vi "Station.Home.Check.vi"(8 "error in (no error)":errorcluster) -> (0 "error out":errorcluster, 1 "Homed?":bool, 2 "Error?":bool, 3 "Statuses":T2[](array[typedef]), 5 "Station Home Status":T1)   [LabVIEW 2016]
uses:
  Station.Home.Status.ctl
  Station.Home.Status.Bits.ctl
  tools/Translator/Translator.Message.ctl
  Drivers/FestoCPX/FestoCPX.State.ctl
  Drivers/V7310/LowLevel/V7310.LaserStatus.ctl
  Drivers/V7310/V7310.Data.Status.State.ctl
  Drivers/Keyence/Keyence.Data.Status.State.ctl
  tools/Translator/Translator.FormatMessage.vi
  tools/Translator/Translator.Global.vi
  Global/ApplicationGlobal.vi
  Sequence/Sequence.Global.vi
  Drivers/FestoCPX/FestoCPX.Global.vi
  Drivers/V7310/LowLevel/V7310.Global.vi
  Drivers/Keyence/LowLevel/Keyence.Global.vi
  Station.Global.vi
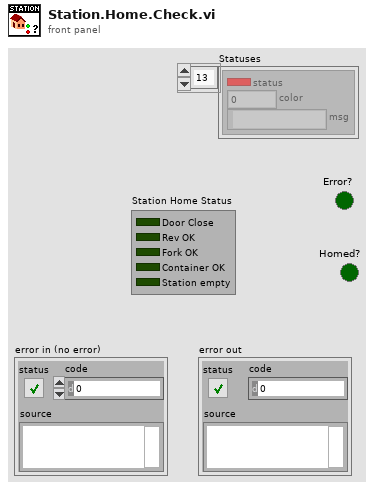
[diagram p1: front panel]
types:
  T1 = typedef "Station.Home.Status.Bits.ctl" = cluster{"Door Close":bool, "Rev OK":bool, "Fork OK":bool, "Container OK":bool, "Station empty":bool}
  T2 = typedef "Station.Home.Status.ctl" = cluster{"status":bool, "color":u32, "msg":string}
  T3 = typedef "Translator.Message.ctl" = enum16{"-", "Event confirmed", "Log out", "Log in", "Shutdown", "Cancel", "Start", "Begin time", "End time", "Duration", "Service Mode", "Ignore Results", "Serial Format", "On", "Off", "OK", "NOK", "NOK %s", "Home", "Work", "Close", "Open", "In progress...", "Missing", "Empty", "Hardware failure", "Initial", "Default", "Total", "Out of range", "Free disk space is below 1GB - contact technician", "Error %d >> %s", "Error %d >> %s >> %s", "Msg %d >> %s", "Laser msg %d %s", "Laser cmd error %s %d", "Laser cmd failed %s", "Laser cmd warning %s", "Laser disconnected", "Laser status %s", "Laser already started", "Laser job unkonwn %s", "Laser job missing %s", "Laser job select failure %s", "Unable to start laser printing (%s)", "Unable to stop laser printing (%s)", "Laser marking aborted", "Laser marking timeout", "Unable to reset Laser Interlock (%s)", "Unable to trigger Laser. Laser not ready (%s)", "Laser job '%s' coordinates not configured", "Starting %s", "Quitting %s", "Configured", "Initializing", "Quitting", "Loading", "Loaded %d results", "Loaded %d events", "Running", "Stopped", "Summary", "Laser", "Do you want to continue?", "Do you want to delete the configuration?", "The configuration is being used by an order. Unable to delete!", "Press confirm button", "Station is not based. Do you want to exit?", "Station requires changeover. Do you want to run the test?", "Test options are not set as default. Do you want to continue?", "Formatting of WabcoNo is disabled. Do you want to continue?", "Product not detected. Do you want to continue?", "Product scan failed. Do you want to continue?", "Calibration", "Log out?", "System", "All", "IDLE", "Translating...%s", "Not found", "Alarm %s", "Run", "Skip", "Abort", "Repeat", "Please wait...", "Database disconnected", "Database disconnected - changeover disabled!", "Login to database successful", "Login to database failed: %d; %s", "Unable to check the product status of reference %d - database disconnected", "Unable to set the product status of reference %d - database disconnected", "Variant file backup %s", "Read variant (%s)", "Result", "Station armed!", "Station requires changeover!", "Select reference number...", "EMERGENCY BUTTON - press Control button", "EMERGENCY DOOR - press Control button", "Resetting Emergency...", "Unable to reset safety circuit - Emergency Button pressed", "Unable to reset safety circuit - Emergency Side Door open", "Station not based", "Station based", "Station not empty", "Station basing...", "No order", "Press Start to begin new order", "Scanning new order", "Order NOK. Correct or scan again", "Order OK. Press Accept", "Order ready", "Revolver incorrect", "Fork incorrect", "Revolver missing", "Revolver empty", "Container missing", "Offline results", "Offline statistics", "Updating statistics %.1f %%", "DMC Configurator", "Door open", "Close the front door", "Press start button", "Done. Open the front door", "Running...", "Running...%.1f %%", "Pause %s", "Pause %s. NOK container missing", "Pause %s. OK container missing", "Pause %s. Revolver empty", "Pause %s. Revolver missing", "Pause %s. Revolver incorrect", "Pause %s. Fork missing", "Pause %s. Fork incorrect", "Pause %s. Too many failures", "Pause %s. Unloading failure", "Pause %s. One slot is not working", "Pause %s. Part order is done. Empty OK container", "Pause %s. Unable to move product to slot", "Pause %s. Unable to move back product pusher", "Pause %s. Unable to lift product", "Pause %s. Unable to move back product lifter", "Pause %s. Unable to move product arm to Work", "Pause %s. Unable to move product arm to NOK", "Pause %s. Unable to move product arm to OK", "Pause %s. Unable to unsuck the NOK product", "Pause %s. Unable to drop the NOK product", "Pause %s. Product OK missing", "Pause %s. Unable to unsuck the OK product", "Pause %s. Unable to drop the OK product", "Stopping...", "File '%s' is missing", "File '%s' is broken", "File '%s' is running", "Log file started (%s)", "Log file ended (%s)", "Log file stopped (%s)", "Log file ignored (%s)", "Log file exported (%s)", "Log file export failed (%s)", "Wrong serial number in log file", "Wrong reference number in log file", "Test steps are missing", "%s = %.3f", "Process param '%s' not found in DB", "Process param '%s' wrong order", "Process param '%s' value %.3f out of limits (%.3f; %.3f)", "Step%d param '%s' not found in DB", "Step%d param '%s' wrong order", "Step%d param '%s' value %.3f out of limits (%.3f; %.3f)", "Step%d EV '%s' not found in DB", "Step%d EV '%s' wrong order", "\"%s\" not found in DB", "\"%s\" wrong order", "\"%s\" value %.3f out of limits (%.3f; %.3f)", "\"%s\" not found in software", "Process init (%s)", "Process started", "Process restarted", "Process run", "Process done", "Process done - remove OK container", "Process aborted", "Process aborted at work", "Process aborted at home", "Process error", "Process error at home", "Process error at work", "Process close", "Process pause", "Process continue", "Process door open", "Process door close", "Process pause at slot %s due to %s", "Select plate from the order to process", "Do you want to start the process?", "Do you want to continue the process?", "There is unfinished order. Do you want to put the new order?", "Product %s %d OK", "Product %s %d NOK", "Unable to unload the slot %s. Product missing in the slot", "Unable to unload the slot %s. Product already in the arm", "Unable to accept the product as OK. Product missing in slot %s", "Unable to accept the product as OK. Product could not drop into the container at slot %s", "Unable to accept the product as NOK. Product could not drop into the container at slot %s", "Scan failed. Error %s", "Scan failed. Scanner disconnected", "Scan failed. Wrong Wabco number %d, limit (%d,%d)", "Scan failed. Wrong serial number %d, limit (%d,%d)", "Scan failed. Wrong date %d, limit (%d,%d)", "Scan failed. Wrong product wabco number %d (expected %d)", "Scan failed. Wrong product serial number %d (expected > 0)", "Scan OK %s", "Scan failed. Unable to determine table position (%s)", "Scan failed. Timeout", "Tune failed. Scanner disconnected", "Tune failed. Timeout", "%s = %d", "%s = %d->%d", "Unable to set %s = %.2f - Air Pressure Inside off", "Unable to set digital output '%s' = %d", "Unable to activate air pressure inside - timeout", "Unable to activate air pressure inside - aborted", "Unable to switch on Air Main Valve - Air Pressure Inlet off", "Unable to switch on Air Main Valve - Door open", "Unable to switch off Air Main Valve - timeout", "Unable to switch off Air Main Valve - aborted", "Unable to rotate Table - timeout", "Unable to rotate Table - aborted", "Unable to rotate Table - Product Move not in Home position", "Unable to rotate Table - Air Pressure Inside off", "Unable to rotate Table - Product Lift A not in Home position", "Unable to rotate Table - Product Lift B not in Home position", "Unable to rotate Table - unlock before movement timeout", "Unable to rotate Table - lock after movement timeout", "Unable to move Table Lock to %s position - timeout", "Unable to move Table Lock to %s position - aborted", "Unable to move Table Lock to %s position - Air Pressure Inside off", "Unable to move Table Lock to %s position - Table not in position", "Unable to move Product Lift A to %s position - timeout", "Unable to move Product Lift B to %s position - timeout", "Unable to move Product Lift A to %s position - aborted", "Unable to move Product Lift B to %s position - aborted", "Unable to move Product Lift A to %s position - Air Pressure Inside off", "Unable to move Product Lift B to %s position - Air Pressure Inside off", "Unable to move Product Lift A to %s position - Table not locked", "Unable to move Product Lift B to %s position - Table not locked", "Unable to move Product Lift A to %s position - Product Arm not in Work position", "Unable to move Product Lift B to %s position - Product Arm not in Work position", "Unable to set Product Suction Gripper %s to %s - timeout", "Unable to set Product Suction Gripper %s to %s - aborted", "Unable to set Product Suction Gripper %s to %s - Air Pressure Inside off", "Unable to set Product Suction Gripper %s to %s - Table slot unkown", "Unable to move Product Arm to %s position - timeout", "Unable to move Product Arm to %s position - aborted", "Unable to move Product Arm to %s position - Air Pressure Inside off", "Unable to move Product Arm to %s position - Product Lift A not in Home position", "Unable to move Product Arm to %s position - Product Lift B not in Home position", "Unable to move Product to %s position - timeout", "Unable to move Product to %s position - aborted", "Unable to move Product to %s position - Air Pressure Inside off", "Unable to move Product to %s position - Table not in position"}
  T4 = typedef "Sequence.Data.ctl" = cluster{"BeginTS":timestamp, "EndTS":timestamp, "State":T5, "Status.Work":T6, "Status.Process":T6, "Status.Home":T6, "Status.Wabco":T6, "Status.Client":T6, "BreakReason":T7, "BreakSource":T8, "DoorLock":bool, "Status.Prod":T9[], "UserAction":T13, "UserData":T14, "Error":errorcluster, "Code":T17, "Rotations":i32, "ProdIdx":i32, "ProdDone":T9[], "PrintedSerials-Wabco":i32[], "PrintedSerials-Client":i32[], "Counters-Wabco":T24, "Counters-Client":T24}
  T5 = typedef "Sequence.State.ctl" = enum16{"Init", "Idle", "Home", "Work", "Run", "Pause"}
  T6 = typedef "Sequence.Step.Status.ctl" = enum16{"-", "Pending", "Running", "Skipped", "Passed", "Failed", "Done", "Error", "Aborted", "Stopped"}
  T7 = typedef "Sequence.Test.BreakReason.ctl" = enum16{"-", "NOK container", "OK container", "Rev empty", "Rev missing", "Rev wrong", "Fork missing", "Fork wrong", "NOK limit", "Unload failure", "Single slot", "Part done", "Err: Prod move work", "Err: Prod move home", "Err: Prod lift work", "Err: Prod lift home", "Err: Prod Arm Work", "Err: Prod Arm NOK", "Err: Prod Arm OK", "Err: Prod NOK suck", "Err: Prod NOK drop", "Err: Prod OK missing", "Err: Prod OK suck", "Err: Prod OK drop"}
  T8 = typedef "Sequence.Test.BreakSource.ctl" = enum16{"-", "A", "B", "A/B"}
  T9 = typedef "Sequence.Test.Status.ctl" = cluster{"Slot":T10, "A":T12, "B":T12}
  T10 = typedef "Sequence.Slot.StatusData.ctl" = cluster{"ID":i32, "Unload":T11, "TS":timestamp, "duration":u32}
  T11 = typedef "Sequence.Test.Unload.Status.ctl" = enum16{"init", "check NOK", "check OK", "wait on NOK", "wait on OK", "wait on Unload", "done"}
  T12 = typedef "Sequence.Prod.StatusData.ctl" = cluster{"status":T6, "pause":T7, "present":bool, "printed":bool, "scanned":bool, "tuned":bool, "removed":bool, "LaserVariables":string[], "ScanerReadOut":string, "path":path, "corners":cluster{"X":i32, "Y":i32}[], "verification":u8}
  T13 = typedef "Sequence.UserActions.ctl" = cluster{"Stop":bool, "Pause":bool, "Next":bool}
  T14 = typedef "Sequence.UserData.ctl" = cluster{"GuiMode":T15, "Test":T16, "ContinueOrder":bool}
  T15 = typedef "Sequence.MainMode.ctl" = enum16{"Process", "Base", "Order", "Manual", "Logs", "Results", "Stats", "DMC Config"}
  T16 = typedef "MainGui.TestOptions.ctl" = cluster{"IgnoreResults":bool, "IgnoreImages":bool, "ServiceMode":bool}
  T17 = typedef "Sequence.Code.Sets.ctl" = cluster{"Ready":bool, "DoubleOrder":bool, "OrderDone":bool, "AllowSingleSlot":bool, "TunedA":bool, "TunedB":bool, "CheckDM":bool, "ThresholdA":u8, "ThresholdB":u8, "Plate":T18, "ImgPath":path, "Variant":T19}
  T18 = typedef "Sequence.PlateType.ctl" = enum16{"Wabco", "Client"}
  T19 = typedef "Logger.Variant.Sets.ctl" = cluster{"State":T20, "ImgPath":path, "WabcoPlate":string, "WabcoProduct":string, "ClientProduct":string, "ClientPlate":string, "TotalQuantity":u16, "OrderQuantity":u16, "Serial":i32, "Wabco":T21, "Client":T21}
  T20 = typedef "Station.Changeover.State.vi" = enum16{"Init", "Scaning", "NOK", "Wait for ack", "Ready"}
  T21 = typedef "Station.Plate.Properties.ctl" = cluster{"LaserJob":string, "AdditionalTxt":string, "FactoryCode":string, "RevID":u8, "ForkID":u8, "FailuresLimit":u16, "GlobalCnt":i32, "Bank":u8, "SerialFormat":T22, "CoordA":T23, "CoordB":T23, "DMCconfig":i32}
  T22 = typedef "Sequence.Code.SerialFormat.ctl" = enum8{"", "6 dig", "7 dig"}
  T23 = typedef "V7310.Job.Sets.ctl" = cluster{"X":dbl, "Y":dbl, "Angle":dbl}
  T24 = typedef "Sequence.Counters.ctl" = cluster{"Expected":u16, "Done":u16, "OK":u16, "NOK":u16, "NOKlimit":u16, "Part":u16, "PartOK":u16}
  T25 = typedef "FestoCPX.Station.ProdPresent.ctl" = cluster{"Slot1":cluster{"A":bool, "B":bool}, "Slot2":cluster{"A":bool, "B":bool}, "Slot3":cluster{"A":bool, "B":bool}, "Slot4":cluster{"A":bool, "B":bool}, "Final":cluster{"A":bool, "B":bool}, "OK":cluster{"A":bool, "B":bool}, "Container":cluster{"OK":bool, "NOK":bool}}
  T26 = typedef "FestoCPX.Station.EmgState.ctl" = cluster{"Button":bool, "SideDoor":bool, "FrontDoor":bool, "DoorSecured":bool}
  T27 = typedef "FestoCPX.Station.RevolverID.ctl" = cluster{"ID":u8, "1":bool, "2":bool, "3":bool, "4":bool, "5":bool}
  T28 = typedef "FestoCPX.State.ctl" = enum16{"First", "Error", "Init", "Run"}
  T29 = typedef "V7310.Data.Status.State.ctl" = enum16{"First", "Init", "Msg", "Error", "Abort", "Idle", "Run"}
  T30 = typedef "V7310.LaserStatus.ctl" = enum16{"-", "FatalError", "Initialize", "KeySwitchOpen", "TimeoutInterlock", "InterlockOpen", "StartUp", "ShutterlockOpen", "Standby", "Ready", "PrepareForMarking", "WaitForTrigger", "Marking"}
  T31 = typedef "Keyence.Data.Status.State.ctl" = enum16{"First", "Init", "Reset", "Idle", "Scan", "Tune"}
  T32 = typedef "FestoCPX.Data.Status.ctl" = cluster{"State":T28, "Conn":refnum<k5>, "TS":timestamp}
  T33 = typedef "V7310.Data.Status.ctl" = cluster{"State":T29, "LaserStatus":T30, "LaserStatusRaw":string, "Ref":refnum<k5>, "RTC TS":timestamp, "Conn TS":timestamp, "Msg":T34[], "JobInUse":string, "Jobs":string[], "Vars":T35[]}
  T34 = typedef "V7310.Message.Data.ctl" = cluster{"ID":i32, "Msg":string}
  T35 = typedef "V7310.Job.Variable.ctl" = cluster{"Name":string, "Value":string}
  T36 = typedef "Keyence.Data.Status.ctl" = cluster{"State":T31, "Ref":refnum<k5>, "Bank":u8, "Version":string, "Model":string, "EndTS":timestamp, "ImgPath":path, "Tuned":bool}
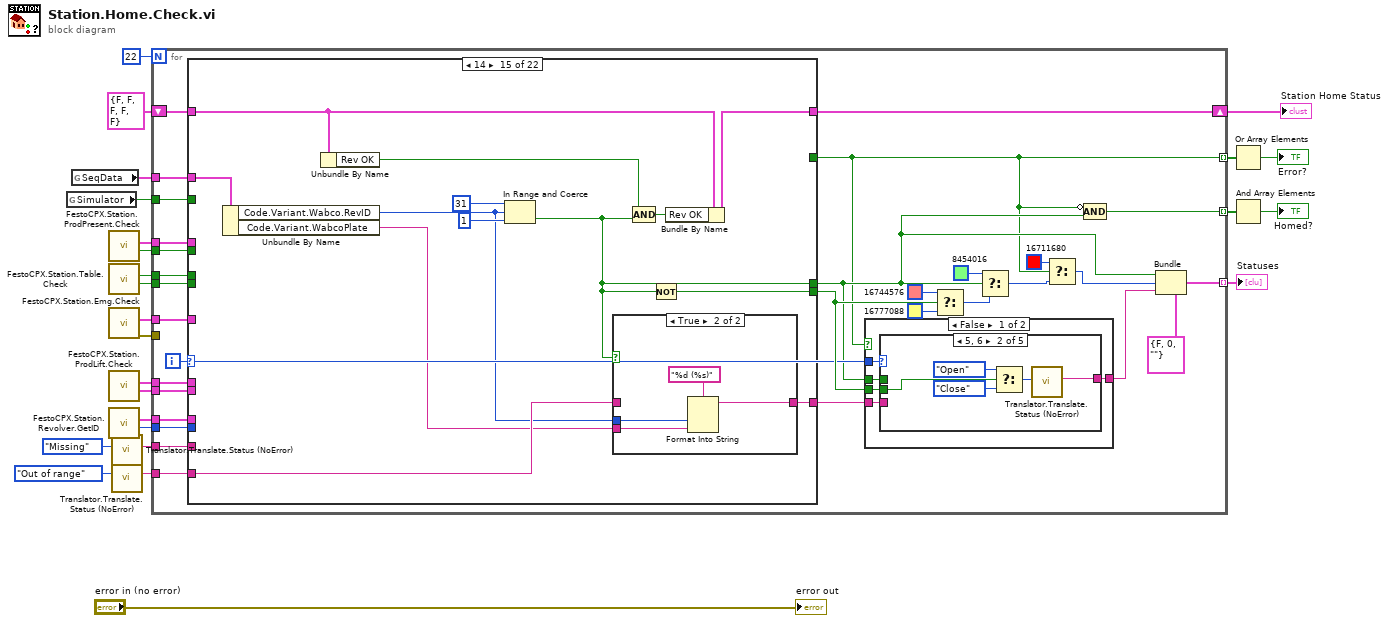
[diagram p0: block diagram]
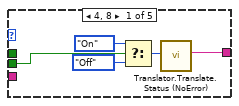
[diagram p2: hidden frame]
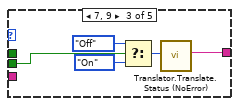
[diagram p3: hidden frame]
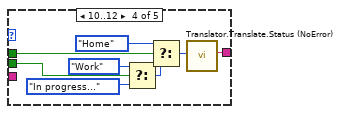
[diagram p4: hidden frame]
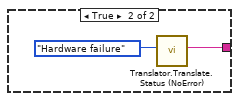
[diagram p6: hidden frame]
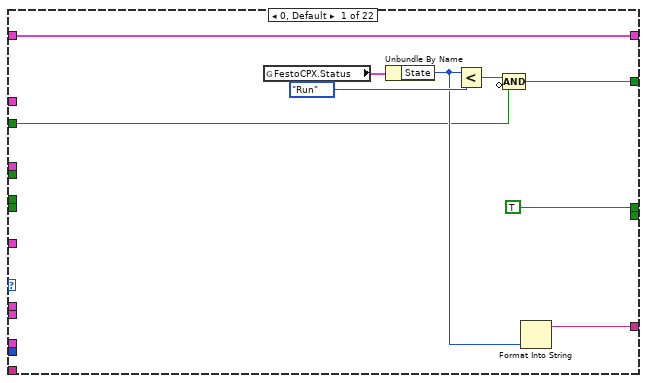
[diagram p7: hidden frame]
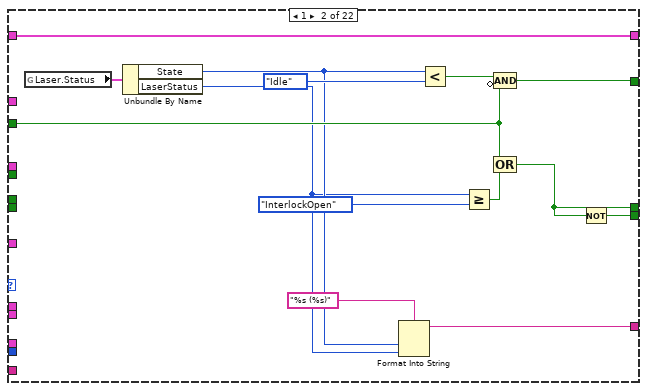
[diagram p8: hidden frame]
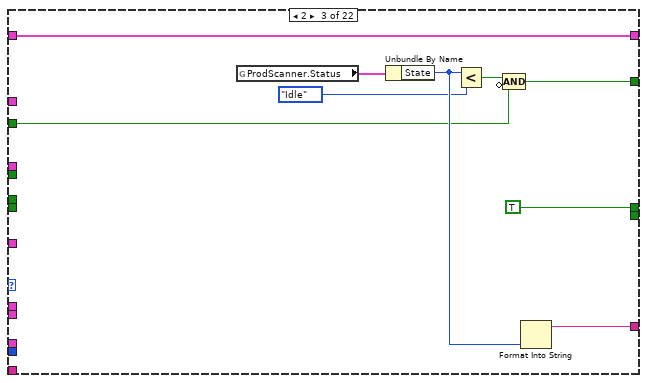
[diagram p9: hidden frame]
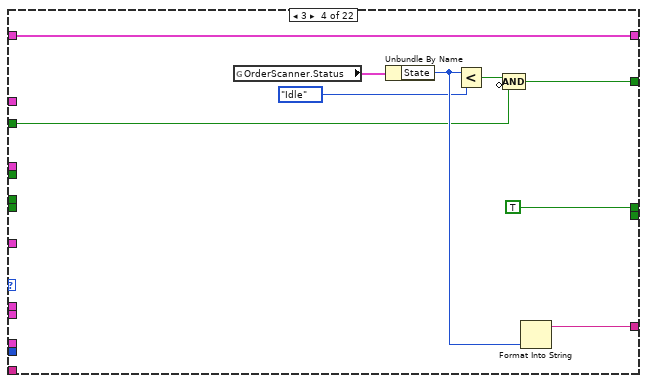
[diagram p10: hidden frame]
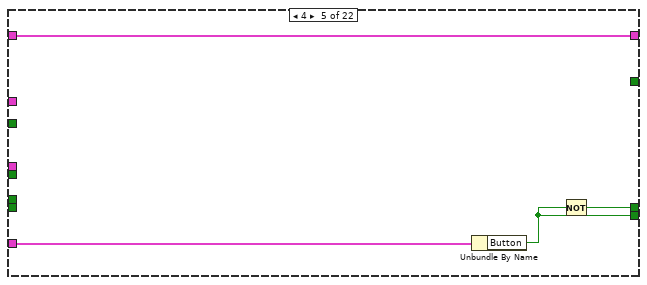
[diagram p11: hidden frame]
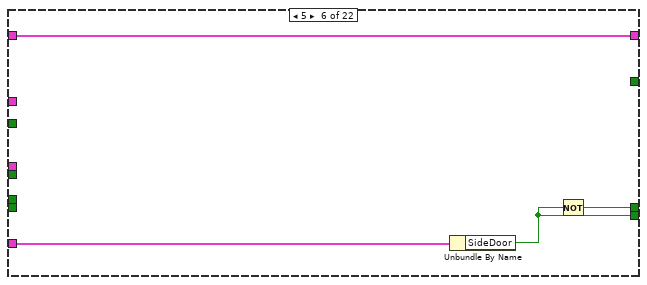
[diagram p12: hidden frame]
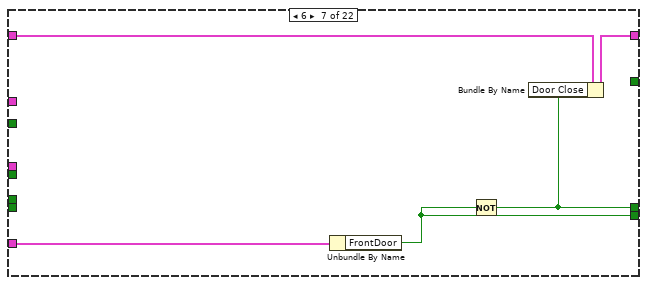
[diagram p13: hidden frame]
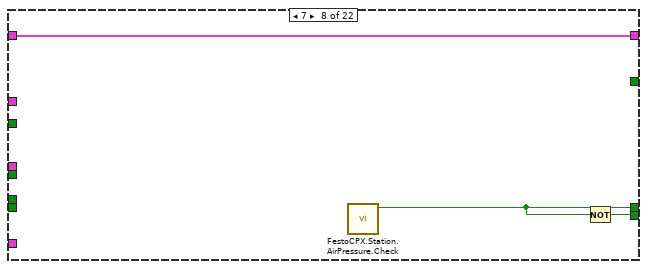
[diagram p14: hidden frame]
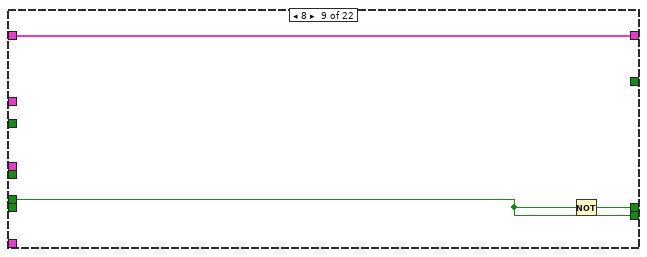
[diagram p15: hidden frame]
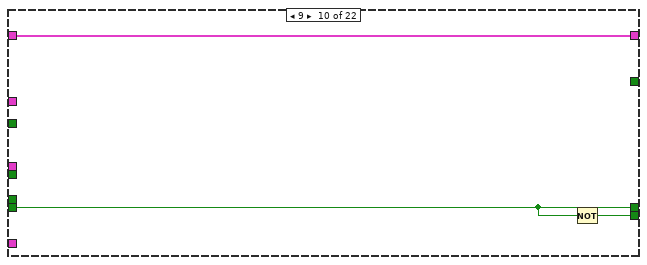
[diagram p16: hidden frame]
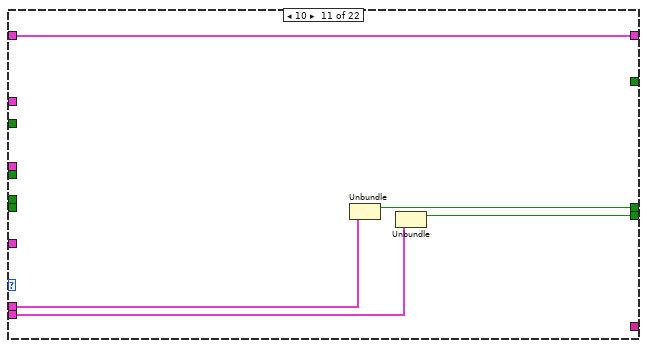
[diagram p17: hidden frame]
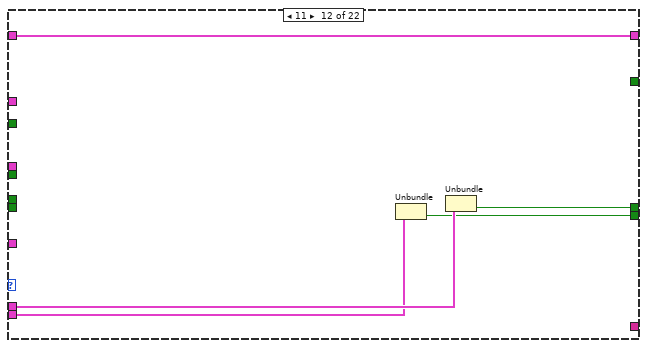
[diagram p18: hidden frame]
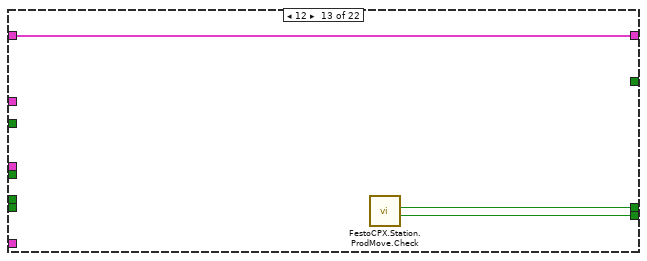
[diagram p19: hidden frame]
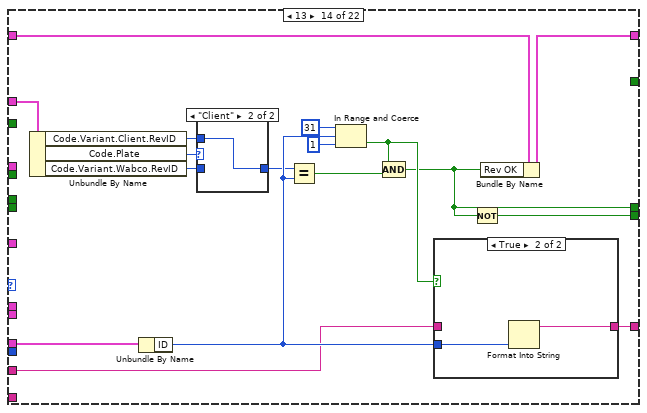
[diagram p20: hidden frame]
diagram:
  n1 = global read "ApplicationGlobal.vi" "Simulator"() -> (w12:bool)
  n2 = global read "Sequence.Global.vi" "SeqData"() -> (w6:T4)
  n3 = call "FestoCPX.Station.ProdPresent.Check.vi"() -> ("table empty (all out)"=w10:bool, "Prod Present"=w11:T25)  [unwired: 6 in, 4 out]
  n4 = call "FestoCPX.Station.Table.Check.vi"() -> ("Table Lock"=w15:bool, "Table Pos"=w16:bool)  [unwired: 9 in, 1 out]
  n5 = call "FestoCPX.Station.Emg.Check.vi"() -> ("error out"=w17:errorcluster, "Emg"=w25:T26)  [unwired: 9 in, 1 out]
  n6 = call "FestoCPX.Station.ProdLift.Check.vi"() -> ("Work"=w13:cluster{"A":bool, "B":bool}, "Home"=w14:cluster{"A":bool, "B":bool})  [unwired: 9 in, 1 out]
  n7 = call "FestoCPX.Station.Revolver.GetID.vi"() -> ("ForkID"=w5:u8, "RevID"=w7:T27)  [unwired: 9 in, 1 out]
  n8 = call "Translator.Translate.Status (NoError).vi"("msg"=Translator.Message."Missing") -> ("Translated Msg"=w1:string)  [unwired: 10 in]
  n9 = call "Translator.Translate.Status (NoError).vi"("msg"=Translator.Message."Out of range") -> ("Translated Msg"=w2:string)  [unwired: 10 in]
  n10 = for {
    N: 22 -> [_]
    tunnel: w25 -> [w54]
    tunnel: [w48] -> w24 mode=indexing
    tunnel: [w43] -> w19 mode=indexing
    tunnel: [w36] -> w20 mode=indexing
    tunnel: w17 -> [_]
    tunnel: w16 -> [w41]
    tunnel: w15 -> [w40]
    tunnel: w14 -> [w39]
    tunnel: w13 -> [w38]
    tunnel: w12 -> [w37]
    tunnel: w11 -> [w35]
    tunnel: w10 -> [w34]
    shift-right: [w32] -> w8
    shift-left: T1 {"Door Close"=FALSE, "Rev OK"=FALSE, "Fork OK"=FALSE, "Container OK"=FALSE, "Station empty"=FALSE} ("Station Home Status") -> [w33]
    tunnel: w7 -> [w31]
    tunnel: w6 -> [w29]
    tunnel: w5 -> [w28]
    tunnel: w2 -> [w26]
    tunnel: w1 -> [w27]
    i -> [w55]
    n11 = case shown="14" w55 {
      tunnel: [_ w110 _ _ w130 w134 w140 w144 w145 w149 w152 w157 w162 w180 w198 w218 w243 w260 w277 w292 w309 w331] -> w56
      tunnel: w54 -> [_ _ _ _ w132 w136 w141 _ _ _ _ _ _ _ _ _ _ _ _ _ _ _]
      tunnel: [TRUE ("Air pressure Inside") w107 TRUE ("Air pressure Inside") TRUE ("Air pressure Inside") w131 w135 w137 w143 w146 w150 w153 w158 w163 w171 w187 w206 w236 w249 w264 w281 w310 w332] -> w42
      tunnel: w41 -> [_ _ _ _ _ _ _ _ w145 _ _ _ _ _ _ _ _ _ _ _ _ _]
      tunnel: w40 -> [_ _ _ _ _ _ _ _ _ w150 _ _ _ _ _ _ _ _ _ _ _ _]
      tunnel: w39 -> [_ _ _ _ _ _ _ _ _ _ w155 w160 _ _ _ _ _ _ _ _ _ _]
      tunnel: w38 -> [_ _ _ _ _ _ _ _ _ _ w154 w159 _ _ _ _ _ _ _ _ _ _]
      tunnel: w37 -> [w90 w101 w115 w124 _ _ _ _ _ _ _ _ _ _ _ _ _ _ _ _ _ _]
      tunnel: [w91 w103 w116 w125 _ _ _ _ _ _ _ _ _ _ _ _ _ _ _ _ _ _] -> w36
      tunnel: w35 -> [_ _ _ _ _ _ _ _ _ _ _ _ _ _ _ _ _ _ _ w285 w329 _]
      tunnel: w34 -> [_ _ _ _ _ _ _ _ _ _ _ _ _ _ _ _ _ _ _ w281 _ _]
      tunnel: w33 -> [w88 w97 w111 w120 w129 w133 w139 w142 w147 w148 w151 w156 w161 w178 w191 w211 w241 w252 w270 w283 w317 w336]
      tunnel: [w88 w97 w111 w120 w129 w133 w138 w142 w147 w148 w151 w156 w161 w177 w196 w216 w240 w258 w275 w282 w316 w336] -> w32
      tunnel: w31 -> [_ _ _ _ _ _ _ _ _ _ _ _ _ w174 _ _ _ _ _ _ _ _]
      tunnel: [w93 w108 w118 w127 _ _ _ _ _ _ _ _ _ w179 w197 w217 w242 w259 w276 w284 w313 w330] -> w30
      tunnel: w29 -> [_ _ _ _ _ _ _ _ _ _ _ _ _ w173 w193 w213 w235 w253 w271 _ _ _]
      tunnel: w28 -> [_ _ _ _ _ _ _ _ _ _ _ _ _ _ _ _ w233 _ _ _ _ _]
      tunnel: w26 -> [_ _ _ _ _ _ _ _ _ _ _ _ _ _ w189 w208 _ w250 w266 _ _ _]
      tunnel: w27 -> [_ _ _ _ _ _ _ _ _ _ _ _ _ w169 _ _ w234 _ _ _ _ _]
      frame 0, Default {
        n12 = global read "FestoCPX.Global.vi" "FestoCPX.Status"() -> (w96:T32)
        n13 = Unbundle By Name(w96) -> ("State"=w94:T28)
        n14 = Less?(x=w94, y=FestoCPX.State."Run") -> (x < y?=w92:bool)
        n15 = Compound Arithmetic op=AND(w92, invert w90) -> (w91:bool)
        n16 = Format Into String(w94) -> (resulting string=w93:string)  [unwired: 3 in, 1 out]
      }
      frame 1 {
        n17 = global read "V7310.Global.vi" "Laser.Status"() -> (w105:T33)
        n18 = Unbundle By Name(w105) -> ("State"=w100:T29, "LaserStatus"=w99:T30)
        n19 = Format Into String(format string="%s (%s)", w100, w99) -> (resulting string=w108:string)  [unwired: 2 in, 1 out]
        n20 = Less?(x=w100, y=V7310.Data.Status.State."Idle") -> (x < y?=w102:bool)
        n21 = Greater Or Equal?(x=w99, y=V7310.LaserStatus."InterlockOpen") -> (x >= y?=w98:bool)
        n22 = Compound Arithmetic op=AND(w102, invert w101) -> (w103:bool)
        n23 = Compound Arithmetic op=OR(w101, w98) -> (w107:bool)
        n24 = Not(x=w107) -> (.not. x?=w110:bool)
      }
      frame 2 {
        n25 = global read "Keyence.Global.vi" "ProdScanner.Status"() -> (w114:T36)
        n26 = Unbundle By Name(w114) -> ("State"=w119:T31)
        n27 = Less?(x=w119, y=Keyence.Data.Status.State."Idle") -> (x < y?=w117:bool)
        n28 = Compound Arithmetic op=AND(w117, invert w115) -> (w116:bool)
        n29 = Format Into String(w119) -> (resulting string=w118:string)  [unwired: 3 in, 1 out]
      }
      frame 3 {
        n30 = global read "Keyence.Global.vi" "OrderScanner.Status"() -> (w123:T36)
        n31 = Unbundle By Name(w123) -> ("State"=w128:T31)
        n32 = Less?(x=w128, y=Keyence.Data.Status.State."Idle") -> (x < y?=w126:bool)
        n33 = Compound Arithmetic op=AND(w126, invert w124) -> (w125:bool)
        n34 = Format Into String(w128) -> (resulting string=w127:string)  [unwired: 3 in, 1 out]
      }
      frame 4 {
        n35 = Unbundle By Name(w132) -> ("Button"=w130:bool)
        n36 = Not(x=w130) -> (.not. x?=w131:bool)
      }
      frame 5 {
        n37 = Unbundle By Name(w136) -> ("SideDoor"=w134:bool)
        n38 = Not(x=w134) -> (.not. x?=w135:bool)
      }
      frame 6 {
        n39 = Unbundle By Name(w141) -> ("FrontDoor"=w140:bool)
        n40 = Not(x=w140) -> (.not. x?=w137:bool)
        n41 = Bundle By Name(cluster=w139, "Door Close"=w137) -> (w138:T1)
      }
      frame 7 {
        n42 = call "FestoCPX.Station.AirPressure.Check.vi"() -> ("Air pressure Inlet"=w143:bool)  [unwired: 8 in, 3 out]
        n43 = Not(x=w143) -> (.not. x?=w144:bool)
      }
      frame 8 {
        n44 = Not(x=w145) -> (.not. x?=w146:bool)
      }
      frame 9 {
        n45 = Not(x=w150) -> (.not. x?=w149:bool)
      }
      frame 10 {
        n46 = Unbundle(w155) -> ("A"=w153:bool)  [unwired: 1 out]
        n47 = Unbundle(w154) -> ("A"=w152:bool)  [unwired: 1 out]
      }
      frame 11 {
        n48 = Unbundle(w159) -> ("B"=w157:bool)  [unwired: 1 out]
        n49 = Unbundle(w160) -> ("B"=w158:bool)  [unwired: 1 out]
      }
      frame 12 {
        n50 = call "FestoCPX.Station.ProdMove.Check.vi"() -> ("Work"=w162:bool, "Home"=w163:bool)  [unwired: 9 in, 1 out]
      }
      frame 13 {
        n51 = Unbundle By Name(w173) -> ("Code.Variant.Client.RevID"=w165:u8, "Code.Plate"=w166:T18, "Code.Variant.Wabco.RevID"=w167:u8)
        n52 = Unbundle By Name(w174) -> ("ID"=w170:u8)
        n53 = case shown="\"Client\"" w166 {
          tunnel: [w181 w182] -> w164
          tunnel: w165 -> [_ w182]
          tunnel: w167 -> [w181 _]
          frame "Wabco", Default {
          }
          frame "Client" {
          }
        }
        n54 = Equal?(x=w164, y=w170) -> (x = y?=w168:bool)
        n55 = In Range and Coerce(upper limit=u8 31, x=w170, lower limit=u8 1) -> (In Range?=w172:bool)  [unwired: 1 out]
        n56 = Compound Arithmetic op=AND(w172, w168) -> (w171:bool)
        n57 = case shown="True" w172 {
          tunnel: [w183 w185] -> w179
          tunnel: w169 -> [w183 _]
          tunnel: w170 -> [_ w184]
          frame False {
          }
          frame True {
            n58 = Format Into String(w184) -> (resulting string=w185:string)  [unwired: 3 in, 1 out]
          }
        }
        n59 = Not(x=w171) -> (.not. x?=w180:bool)
        n60 = Bundle By Name(cluster=w178, "Rev OK"=w171) -> (w177:T1)
      }
      frame 14 {
        n61 = Unbundle By Name(w193) -> ("Code.Variant.Wabco.RevID"=w188:u8, "Code.Variant.WabcoPlate"=w186:string)
        n62 = Unbundle By Name(w191) -> ("Rev OK"=w190:bool)
        n63 = In Range and Coerce(upper limit=u8 31, x=w188, lower limit=u8 1) -> (In Range?=w187:bool)  [unwired: 1 out]
        n64 = case shown="True" w187 {
          tunnel: [w199 w203] -> w197
          tunnel: w189 -> [w199 _]
          tunnel: w188 -> [_ w202]
          tunnel: w186 -> [_ w200]
          frame False {
          }
          frame True {
            n65 = Format Into String(format string="%d (%s)", w202, w200) -> (resulting string=w203:string)  [unwired: 2 in, 1 out]
          }
        }
        n66 = Compound Arithmetic op=AND(w190, w187) -> (w192:bool)
        n67 = Not(x=w187) -> (.not. x?=w198:bool)
        n68 = Bundle By Name(cluster=w191, "Rev OK"=w192) -> (w196:T1)
      }
      frame 15 {
        n69 = Unbundle By Name(w213) -> ("Code.DoubleOrder"=w204:bool, "Code.Variant.Client.RevID"=w207:u8, "Code.Variant.ClientPlate"=w205:string)
        n70 = Unbundle By Name(w211) -> ("Rev OK"=w209:bool)
        n71 = In Range and Coerce(upper limit=u8 31, x=w207, lower limit=u8 1) -> (In Range?=w212:bool)  [unwired: 1 out]
        n72 = Compound Arithmetic op=OR(invert w204, w212) -> (w206:bool)
        n73 = case shown="True" w206 {
          tunnel: w207 -> [_ w223]
          tunnel: [w219 w222] -> w217
          tunnel: w208 -> [w219 _]
          tunnel: w205 -> [_ w221]
          tunnel: w204 -> [_ w220]
          frame False {
          }
          frame True {
            n74 = case shown="True" w220 {
              tunnel: w223 -> [_ w227]
              tunnel: [_ w226] -> w222
              tunnel: w221 -> [_ w225]
              frame False {
              }
              frame True {
                n75 = Format Into String(format string="%d (%s)", w227, w225) -> (resulting string=w226:string)  [unwired: 2 in, 1 out]
              }
            }
          }
        }
        n76 = Compound Arithmetic op=AND(w209, w206) -> (w210:bool)
        n77 = Not(x=w206) -> (.not. x?=w218:bool)
        n78 = Bundle By Name(cluster=w211, "Rev OK"=w210) -> (w216:T1)
      }
      frame 16 {
        n79 = Unbundle By Name(w235) -> ("Code.Variant.Client.ForkID"=w229:u8, "Code.Plate"=w231:T18, "Code.Variant.Wabco.ForkID"=w228:u8)
        n80 = case shown="\"Wabco\", Default" w231 {
          tunnel: [w244 w245] -> w230
          tunnel: w229 -> [_ w245]
          tunnel: w228 -> [w244 _]
          frame "Wabco", Default {
          }
          frame "Client" {
          }
        }
        n81 = Equal?(x=w230, y=w233) -> (x = y?=w232:bool)
        n82 = In Range and Coerce(upper limit=u8 3, x=w233, lower limit=u8 1) -> (In Range?=w239:bool)  [unwired: 1 out]
        n83 = Compound Arithmetic op=AND(w239, w232) -> (w236:bool)
        n84 = case shown="True" w239 {
          tunnel: w233 -> [_ w248]
          tunnel: [w246 w247] -> w242
          tunnel: w234 -> [w246 _]
          frame False {
          }
          frame True {
            n85 = Format Into String(w248) -> (resulting string=w247:string)  [unwired: 3 in, 1 out]
          }
        }
        n86 = Not(x=w236) -> (.not. x?=w243:bool)
        n87 = Bundle By Name(cluster=w241, "Fork OK"=w236) -> (w240:T1)
      }
      frame 17 {
        n88 = Unbundle By Name(w253) -> ("Code.Variant.Wabco.ForkID"=w255:u8)
        n89 = Unbundle By Name(w252) -> ("Fork OK"=w251:bool)
        n90 = In Range and Coerce(upper limit=u8 3, x=w255, lower limit=u8 1) -> (In Range?=w249:bool)  [unwired: 1 out]
        n91 = Compound Arithmetic op=AND(w251, w249) -> (w254:bool)
        n92 = case shown="False" w249 {
          tunnel: w255 -> [_ w263]
          tunnel: [w261 w262] -> w259
          tunnel: w250 -> [w261 _]
          frame False {
          }
          frame True {
            n93 = Format Into String(w263) -> (resulting string=w262:string)  [unwired: 3 in, 1 out]
          }
        }
        n94 = Not(x=w249) -> (.not. x?=w260:bool)
        n95 = Bundle By Name(cluster=w252, "Fork OK"=w254) -> (w258:T1)
      }
      frame 18 {
        n96 = Unbundle By Name(w271) -> ("Code.DoubleOrder"=w267:bool, "Code.Variant.Client.ForkID"=w265:u8)
        n97 = Unbundle By Name(w270) -> ("Fork OK"=w269:bool)
        n98 = In Range and Coerce(upper limit=u8 3, x=w265, lower limit=u8 1) -> (In Range?=w268:bool)  [unwired: 1 out]
        n99 = Compound Arithmetic op=OR(invert w267, w268) -> (w264:bool)
        n100 = Compound Arithmetic op=AND(w269, w264) -> (w272:bool)
        n101 = case shown="True" w264 {
          tunnel: [w278 w280] -> w276
          tunnel: w266 -> [w278 _]
          tunnel: w265 -> [_ w279]
          frame False {
          }
          frame True {
            n102 = Format Into String(w279) -> (resulting string=w280:string)  [unwired: 3 in, 1 out]
          }
        }
        n103 = Not(x=w264) -> (.not. x?=w277:bool)
        n104 = Bundle By Name(cluster=w270, "Fork OK"=w272) -> (w275:T1)
      }
      frame 19 {
        n105 = Cluster To Array(cluster=w285) -> (array=w291:cluster{"OK":bool, "NOK":bool}[])
        n106 = for {
          tunnel: w291 -> [w298] mode=indexing
          tunnel: string[] ["Slot1", "Slot2", "Slot3", "Slot4", "Final", "Output"] -> [w297] mode=indexing
          tunnel: [w296] -> w289 mode=indexing
          w294 = ""
          n107 = Unbundle(w298) -> ("OK"=w293:bool, "NOK"=w295:bool)
          n108 = Select(t="A", s=w293, f=w294) -> (s? t:f=w303:string)
          n109 = Select(t="B", s=w295, f=w294) -> (s? t:f=w302:string)
          n110 = Compound Arithmetic op=OR(w293, w295) -> (w304:bool)
          n111 = Format Into String(format string=":%s%s", initial string=w297, w303, w302) -> (resulting string=w300:string)  [unwired: 1 in, 1 out]
          n112 = Select(t=w300, s=w304, f="") -> (s? t:f=w296:string)
        }
        n113 = call <vilib>:"Space Constant.vi"() -> ("String"=w288:string)
        n114 = Array To Spreadsheet String(delimiter (Tab)=w288, array=w289, 3:"%s" ("format string")) -> (spreadsheet string=w286:string)
        n115 = call <vilib>:"Trim Whitespace.vi"("string"=w286) -> ("trimmed string"=w284:string)  [unwired: 1 in]
        n116 = Bundle By Name(cluster=w283, "Station empty"=w281) -> (w282:T1)
        n117 = Not(x=w281) -> (.not. x?=w292:bool)
      }
      frame 20 {
        w326 = ""
        n118 = Unbundle By Name(w329) -> ("Container.OK"=w319:bool, "Container.NOK"=w318:bool)
        n119 = Select(t=w326, s=w319, f="OK") -> (s? t:f=w321:string)
        n120 = Select(t=w326, s=w318, f="NOK") -> (s? t:f=w322:string)
        n121 = Build Array(w321, w322) -> (w320:string[])
        n122 = Compound Arithmetic op=AND(w319, w318) -> (w310:bool)
        n123 = call <vilib>:"Space Constant.vi"() -> ("String"=w325:string)
        n124 = Array To Spreadsheet String(delimiter (Tab)=w325, array=w320, 3:"%s" ("format string")) -> (spreadsheet string=w323:string)
        n125 = call "Translator.Translate.Status (NoError).vi"("msg"=Translator.Message."Missing") -> ("Translated Msg"=w312:string)  [unwired: 10 in]
        n126 = call <vilib>:"Trim Whitespace.vi"("string"=w323) -> ("trimmed string"=w311:string)  [unwired: 1 in]
        n127 = call <vilib>:"Space Constant.vi"() -> ("String"=w314:string)
        n128 = Bundle By Name(cluster=w317, "Container OK"=w310) -> (w316:T1)
        n129 = Concatenate Strings(w312, w314, w311) -> (w307:string)
        n130 = Not(x=w310) -> (.not. x?=w309:bool)
        n131 = Select(t="", s=w310, f=w307) -> (s? t:f=w313:string)
      }
      frame 21 {
        n132 = global read "Station.Global.vi" "ScannerSlot"() -> (w335:i32)
        n133 = Format Into String(w335) -> (resulting string=w330:string)  [unwired: 3 in, 1 out]
        n134 = In Range and Coerce(upper limit=4 ("lower limit"), x=w335, lower limit=1) -> (In Range?=w332:bool)  [unwired: 1 out]
        n135 = Not(x=w332) -> (.not. x?=w331:bool)
      }
    }
    n136 = case shown="False" w36 {
      tunnel: w56 -> [w61 _]
      tunnel: w55 -> [w60 _]
      tunnel: w30 -> [w59 _]
      tunnel: [w58 w87] -> w49
      tunnel: w42 -> [w57 _]
      frame False {
        n137 = case shown="5, 6" w60 {
          tunnel: w57 -> [_ _ _ w83 _]
          tunnel: w61 -> [w64 w69 w74 w79 _]
          tunnel: [w62 w67 w72 w77 w85] -> w58
          tunnel: w59 -> [_ _ _ _ w85]
          frame 4, 8 {
            n138 = Select(t=Translator.Message."On" ("msg"), s=w64, f=Translator.Message."Off" ("msg")) -> (s? t:f=w63:T3)
            n139 = call "Translator.Translate.Status (NoError).vi"("msg"=w63) -> ("Translated Msg"=w62:string)  [unwired: 10 in]
          }
          frame 5, 6 {
            n140 = Select(t=Translator.Message."Open" ("msg"), s=w69, f=Translator.Message."Close" ("msg")) -> (s? t:f=w68:T3)
            n141 = call "Translator.Translate.Status (NoError).vi"("msg"=w68) -> ("Translated Msg"=w67:string)  [unwired: 10 in]
          }
          frame 7, 9 {
            n142 = Select(t=Translator.Message."Off" ("msg"), s=w74, f=Translator.Message."On" ("msg")) -> (s? t:f=w73:T3)
            n143 = call "Translator.Translate.Status (NoError).vi"("msg"=w73) -> ("Translated Msg"=w72:string)  [unwired: 10 in]
          }
          frame 10..12 {
            n144 = Select(t=Translator.Message."Work" ("msg"), s=w79, f=Translator.Message."In progress..." ("msg")) -> (s? t:f=w84:T3)
            n145 = Select(t=Translator.Message."Home" ("msg"), s=w83, f=w84) -> (s? t:f=w78:T3)
            n146 = call "Translator.Translate.Status (NoError).vi"("msg"=w78) -> ("Translated Msg"=w77:string)  [unwired: 10 in]
          }
          frame Default {
          }
        }
      }
      frame True {
        n147 = call "Translator.Translate.Status (NoError).vi"("msg"=Translator.Message."Hardware failure") -> ("Translated Msg"=w87:string)  [unwired: 10 in]
      }
    }
    n148 = Select(t=u32 16744576, s=w56, f=u32 16777088) -> (s? t:f=w52:u32)
    n149 = Select(t=u32 8454016, s=w42, f=w52) -> (s? t:f=w46:u32)
    n150 = Select(t=u32 16711680, s=w36, f=w46) -> (s? t:f=w44:u32)
    n151 = Compound Arithmetic op=AND(invert w36, w42) -> (w43:bool)
    n152 = Bundle(cluster=T2 {"status"=FALSE, "color"=0, "msg"=""} ("HomeStatus"), "status"=w42, "color"=w44, "msg"=w49) -> (w48:T2)
  }
  "Statuses" <- w24
  "Station Home Status" <- w8
  n153 = Or Array Elements(Boolean array=w20) -> (logical OR=→"Error?":bool)
  n154 = And Array Elements(Boolean array=w19) -> (logical AND=→"Homed?":bool)
  "error out" <- "error in (no error)"
